vi "23_1.vi"() -> ()   [LabVIEW 2020]
panel:
  out "concatenated string":string="69852437"
  in  "Moves":i32=100
  in  "Switch":bool
  in  "Input":string="925176834"
  in  "Input Test":string="389125467"
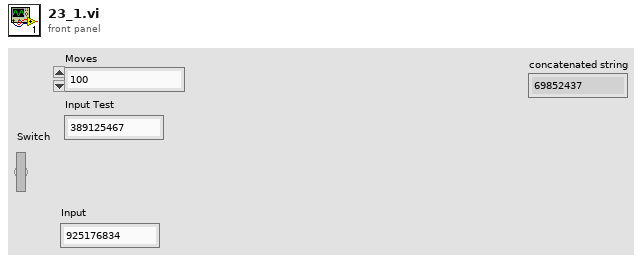
[diagram p1: front panel]
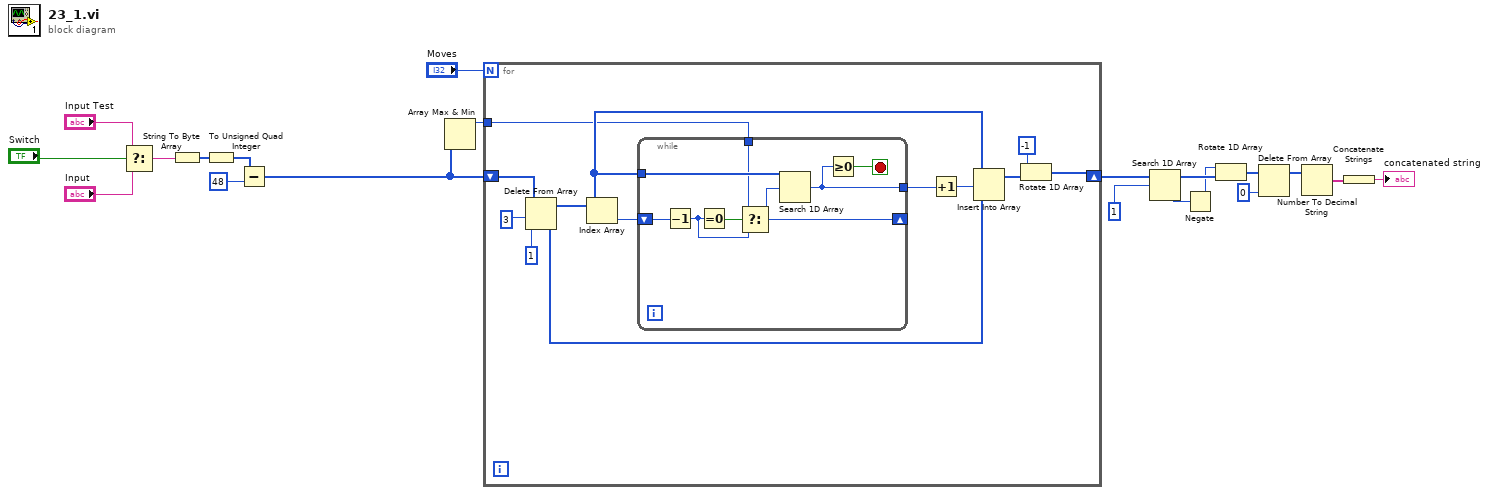
[diagram p0: block diagram]
diagram:
  n1 = Select(t="Input Test", s="Switch", f="Input") -> (s? t:f=w16:string)
  n2 = String To Byte Array(string=w16) -> (unsigned byte array=w15:u8[])
  n3 = To Unsigned Quad Integer(1:w15) -> (0:w6:u64[])
  n4 = Subtract(x=w6, y=u64 48) -> (x-y=w11:u64[])
  n5 = Array Max & Min(array=w11) -> (max value=w10:u64)  [unwired: 3 out]
  n6 = for {
    N: "Moves" -> [_]
    shift-right: [w22] -> w9
    shift-left: w11 -> [w31]
    tunnel: w10 -> [w20]
    n7 = Delete From Array(array=w31, length=3, index=1) -> (deleted portion=w25:u64[], array with subset deleted=w28:u64[])
    n8 = Index Array(array=w28) -> (element=w24:u64)  [unwired: 1 in]
    n9 = while {
      tunnel: w28 -> [w36]
      shift-right: [w34] -> _
      shift-left: w24 -> [w39]
      tunnel: [w33] -> w27
      tunnel: w20 -> [w32]
      stop <- w35 stop-if-true
      n10 = Decrement(x=w39) -> (x-1=w37:u64)
      n11 = Equal To 0?(x=w37) -> (x = 0?=w38:bool)
      n12 = Select(t=w32, s=w38, f=w37) -> (s? t:f=w34:u64)
      n13 = Search 1D Array(1D array=w36, element=w34) -> (index of element=w33:i32)  [unwired: 1 in]
      n14 = Greater Or Equal To 0?(x=w33) -> (x >= 0?=w35:bool)
    }
    n15 = Increment(x=w27) -> (x+1=w26:i32)
    n16 = Insert Into Array(array=w28, index=w26, new element=w25) -> (w23:u64[])
    n17 = Rotate 1D Array(1:w23, 2:-1 ("n")) -> (0:w22:u64[])
  }
  n18 = Search 1D Array(1D array=w9, element=u64 1) -> (index of element=w8:i32)  [unwired: 1 in]
  n19 = Negate(x=w8) -> (-x=w7:i32)
  n20 = Rotate 1D Array(1:w9, 2:w7) -> (0:w5:u64[])
  n21 = Delete From Array(array=w5, index=0) -> (array with subset deleted=w3:u64[])  [unwired: 1 in, 1 out]
  n22 = Number To Decimal String(number=w3) -> (decimal integer string=w4:string[])  [unwired: 1 in]
  n23 = Concatenate Strings(w4) -> (→"concatenated string":string)
